vi "Quake ASEE Demo With Gs.vi"() -> ()   [LabVIEW 2011]
panel:
  in  "stop (F) 2":bool caption="stop (F)"
  out "appended array":bool[](array[boolean])
  out "Waveform Chart":waveform(dbl)[](graph)
  in  "Axis":u16(ring)=3 items=["X"=1, "Y"=2, "Z"=3]
  in  "Axis":u16(ring)=3 items=["X"=1, "Y"=2, "Z"=3]
  out "Peak Reading A (g)":dbl format="%#.4g"
  out "Peak Reading B (g)":dbl format="%#.4g"
  in  "%Full Scale":dbl(slide)=18.954248366013072 scale=0.0..100.0
  in  "stop (F)":bool
  # "myQuake Control and Data Collection"
  # "Accelerometer A"
  # "Accelerometer B"
  # "Motor Control"
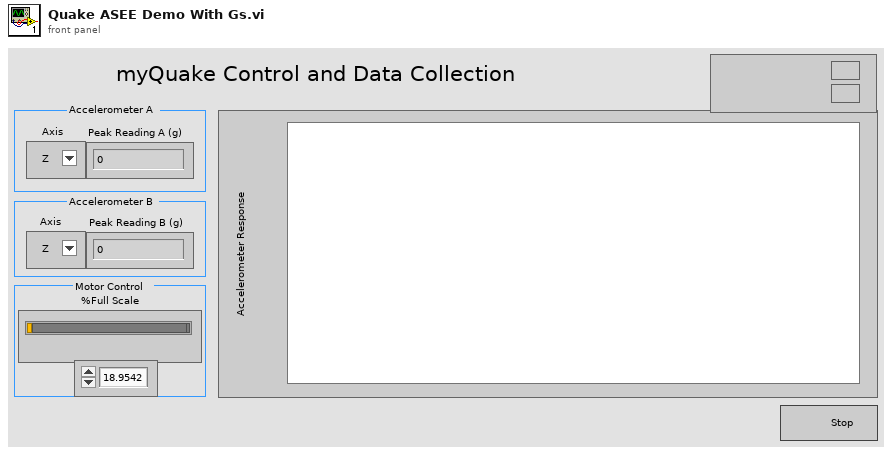
[diagram p1: front panel]
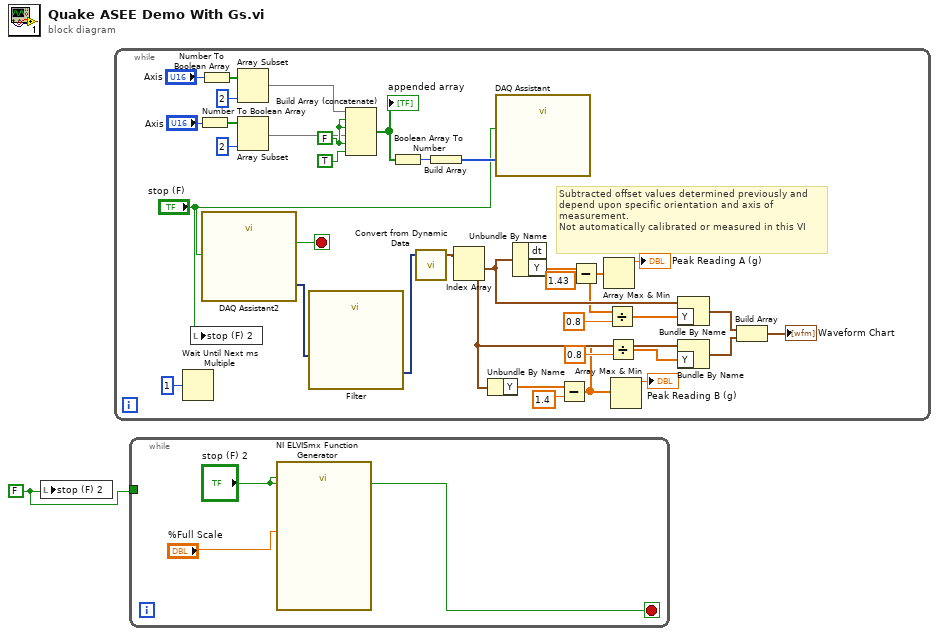
[diagram p0: block diagram]
diagram:
  w1 = FALSE
  n1 = local write "stop (F) 2"(w1) -> ()
  n2 = while {
    stop <- w37 stop-if-true
    w22 = FALSE
    # "Subtracted offset values determined previously and depend upon specific orientation and axis of measurement.\nNot automatically calibrated or measured in this VI"
    n3 = Wait Until Next ms Multiple(millisecond multiple=u32 1) -> ()  [unwired: 1 out]
    n4 = local write "stop (F) 2"("stop (F)") -> ()
    n5 = Number To Boolean Array(number="Axis") -> (Boolean array=w26:bool[])
    n6 = Number To Boolean Array(number="Axis") -> (Boolean array=w30:bool[])
    n7 = call "DAQ Assistant2"("stop (F)"="stop (F)") -> ("data"=w34:dynamicdata, "stopped"=w37:bool)  [unwired: 15 in, 2 out]
    n8 = Array Subset(array=w30, length=2) -> (w29:bool[])  [unwired: 1 in]
    n9 = Array Subset(array=w26, length=2) -> (w21:bool[])  [unwired: 1 in]
    n10 = call "Filter"("Signal"=w34) -> ("Filtered Signal"=w20:dynamicdata)  [unwired: 9 in, 1 out]
    n11 = Build Array (concatenate)(w29, w22, w22, w21, w22, TRUE) -> (w33:bool[])
    "appended array" <- w33
    n12 = Boolean Array To Number(Boolean array=w33) -> (number=w36:u32)
    n13 = call "Convert from Dynamic Data"("Dynamic Data Type"=w20) -> ("Array of Waveform"=w19:waveform(dbl)[])  [unwired: 3 in]
    n14 = Build Array(w36) -> (w35:u32[])
    n15 = Index Array(array=w19) -> (element #1=w11:waveform(dbl), element #2=w12:waveform(dbl))  [unwired: 2 in]
    n16 = Unbundle By Name(w12) -> ("Y"=w13:dbl[])
    n17 = call "DAQ Assistant"("data"=w35, "stop (T)"="stop (F)") -> ()  [unwired: 16 in, 2 out]
    n18 = Unbundle By Name(w11) -> ("Y"=w18:dbl[])  [unwired: 1 out]
    n19 = Subtract(x=w13, y=1.4) -> (x-y=w4:dbl[])
    n20 = Subtract(x=w18, y=1.43) -> (x-y=w8:dbl[])
    n21 = Array Max & Min(array=w8) -> (max value=→"Peak Reading A (g)":dbl)  [unwired: 3 out]
    n22 = Divide(x=w8, y=0.8) -> (x/y=w2:dbl[])
    n23 = Divide(x=w4, y=0.8) -> (x/y=w5:dbl[])
    n24 = Array Max & Min(array=w4) -> (max value=→"Peak Reading B (g)":dbl)  [unwired: 3 out]
    n25 = Bundle By Name(cluster=w11, "Y"=w2) -> (w10:waveform(dbl))
    n26 = Bundle By Name(cluster=w12, "Y"=w5) -> (w9:waveform(dbl))
    n27 = Build Array(w10, w9) -> (→"Waveform Chart":waveform(dbl)[])
  }
  n28 = while {
    tunnel: w1 -> [_]
    stop <- "stop (F) 2" stop-if-true
    n29 = call "NI ELVISmx Function Generator"("Stop"="stop (F) 2", "Duty Cycle (%)"="%Full Scale") -> ()  [unwired: 16 in, 2 out]
  }
